vi "Sequence.vi"() -> ()   [LabVIEW 2016]
uses:
  PID2ChanGlobals.vi
  Globals/LJ_Handles_Global.vi
  <vilib>/Utility/file.llb/Write Delimited Spreadsheet (DBL).vi
panel:
  out "path":path=path "_run0.txt"
  in  "Run":dbl=102.0
  out "Recording Time":dbl=30.0
  out "Measured Ratio":dbl[](graph)
  in  "file path (dialog if empty)":path=path "E:/maggot images/Jacob/20170911/Fluorescein_Test_Step2a_run"
  in  "Add Ctrl?":bool
  in  "Setpoint":dbl[](array[numeric])=[0.9, 0.8, 0.7, 0.6, 0.5, 0.4, 0.3, 0.2, 0.1]
  in  "Time":dbl[](array[numeric])=[30.0, 30.0, 30.0, 30.0, 30.0, 30.0, 30.0, 30.0, 30.0]
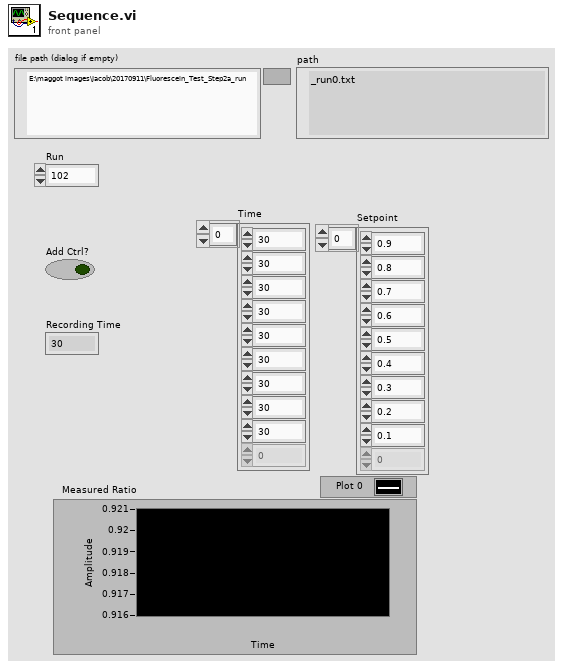
[diagram p1: front panel]
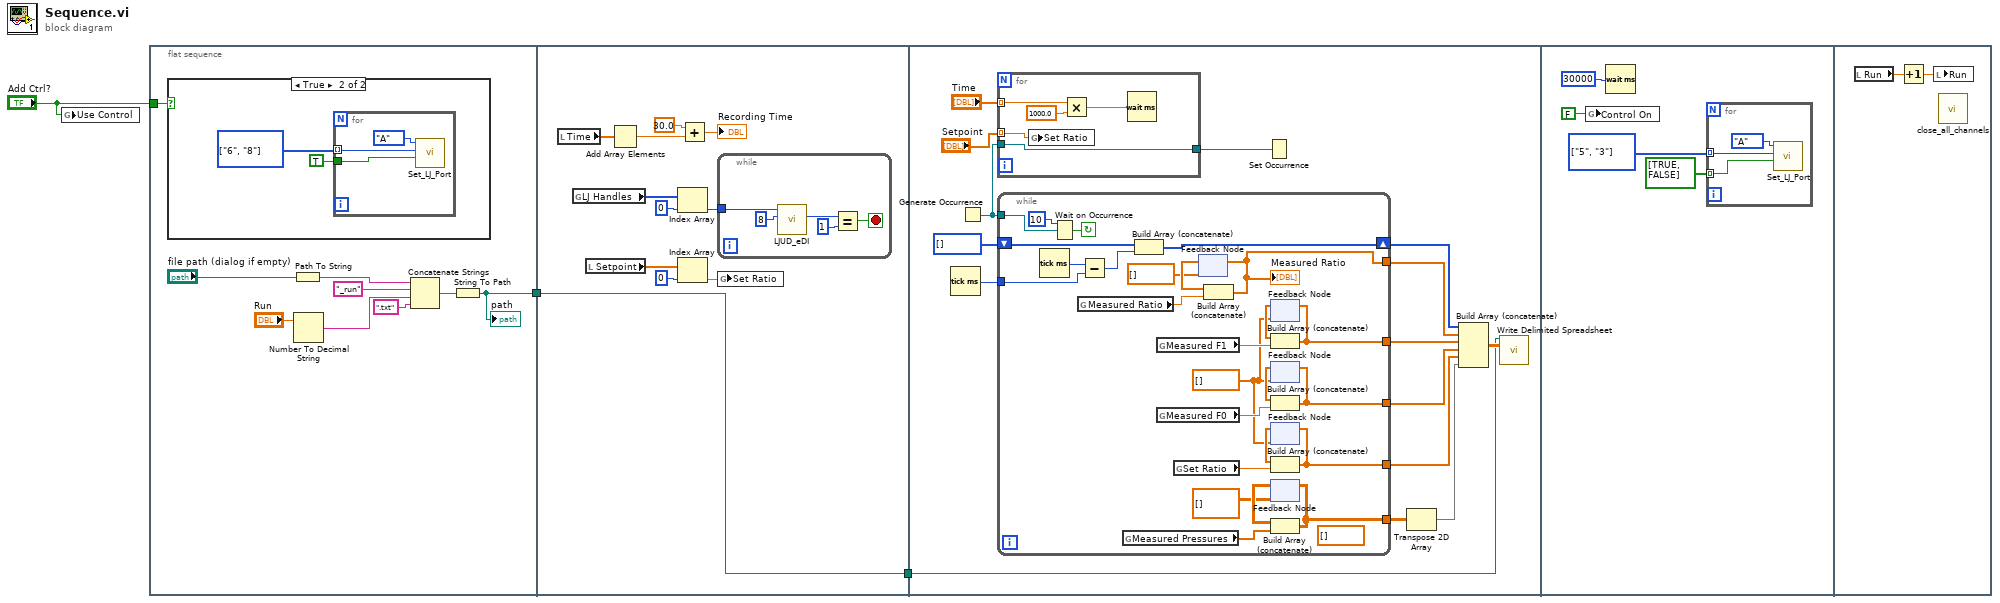
[diagram p0: block diagram]
diagram:
  n1 = global write "PID2ChanGlobals.vi" "Use Control"("Add Ctrl?") -> ()
  n2 = flat-sequence {
    tunnel: "Add Ctrl?" -> [w12]
    tunnel: [w4] -> w1
    tunnel: [w18] -> w2
    tunnel: w1 -> [w18]
    tunnel: w2 -> [w36]
    frame #0 {
      n3 = case shown="True" w12 {
        frame False {
        }
        frame True {
          w13 = enum16{"1", "2", "3", "4", "5", "6", "7", "8"}[] [enum."6", enum."8"] items=["1", "2", "3", "4", "5", "6", "7", "8"]
          n4 = for {
            tunnel: TRUE ("State") -> [w17]
            tunnel: w13 -> [w16] mode=indexing
            n5 = call "Set_LJ_Port.vi"("State"=w17, "Channel"=w16, "Flowboard"=enum16{"A", "B", "C"}."A") -> ()  [unwired: 8 in, 1 out]
          }
        }
      }
      n6 = Path To String(path="file path (dialog if empty)") -> (string=w7:string)
      n7 = Number To Decimal String(number="Run") -> (decimal integer string=w8:string)  [unwired: 1 in]
      n8 = Concatenate Strings(w7, "_run" ("string"), w8, ".txt" ("string")) -> (w5:string)
      n9 = String To Path(string=w5) -> (path=w4:path)
      "path" <- w4
    }
    frame #1 {
      n10 = local read "Time"() -> (w22:dbl[])
      n11 = global read "LJ_Handles_Global.vi" "LJ Handles"() -> (w27:i32[])
      n12 = local read "Setpoint"() -> (w24:dbl[])
      n13 = Add Array Elements(numeric array=w22) -> (sum=w21:dbl)
      n14 = Index Array(array=w27, index=0) -> (element=w26:i32)
      n15 = Index Array(array=w24, index=0) -> (element=w23:dbl)
      n16 = Add(x=30.0, y=w21) -> (x+y=→"Recording Time":dbl)
      n17 = while {
        tunnel: w26 -> [w33]
        stop <- w29 stop-if-true
        n18 = call "LJUD_eDI.vi"("Channel"=8, "Handle In"=w33) -> ("State"=w31:i32)  [unwired: 7 in, 2 out]
        n19 = Equal?(x=w31, y=1) -> (x = y?=w29:bool)
      }
      n20 = global write "PID2ChanGlobals.vi" "Set Ratio"(w23) -> ()
    }
    frame #2 {
      n21 = Tick Count (ms)() -> (millisecond timer value=w43:u32)
      n22 = Generate Occurrence() -> (w45:refnum<k4>)
      n23 = for {
        tunnel: "Time" -> [w76] mode=indexing
        tunnel: "Setpoint" -> [w78] mode=indexing
        tunnel: w45 -> [w79]
        tunnel: [w79] -> w46
        n24 = global write "PID2ChanGlobals.vi" "Set Ratio"(w78) -> ()
        n25 = Multiply(x=w76, y=1000.0) -> (x*y=w75:dbl)
        n26 = Wait (ms)(milliseconds to wait=w75) -> ()  [unwired: 1 out]
      }
      n27 = while {
        tunnel: w45 -> [w73]
        tunnel: [w70] -> w42
        tunnel: w43 -> [w68]
        tunnel: [w62] -> w40
        tunnel: [w59] -> w39
        tunnel: [w56] -> w38
        tunnel: [w53] -> w37
        shift-right: [w69] -> w41
        shift-left: u32[] [] -> [w50]
        stop <- w74 continue-if-true
        (unwired) dbl[] []
        w52 = dbl[] []
        n28 = Tick Count (ms)() -> (millisecond timer value=w67:u32)
        n29 = Wait on Occurrence(2:w73, 3:10 ("ms timeout (-1)")) -> (0:w74:bool)  [unwired: 1 in]
        n30 = global read "PID2ChanGlobals.vi" "Measured Ratio"() -> (w71:dbl)
        n31 = Subtract(x=w67, y=w68) -> (x-y=w66:u32)
        n32 = global read "PID2ChanGlobals.vi" "Measured Pressures"() -> (w55:dbl[])
        n33 = Build Array (concatenate)(w50, w66) -> (w69:u32[])
        n34 = global read "PID2ChanGlobals.vi" "Measured F1"() -> (w64:dbl)
        n35 = global read "PID2ChanGlobals.vi" "Measured F0"() -> (w61:dbl)
        n36 = global read "PID2ChanGlobals.vi" "Set Ratio"() -> (w58:dbl)
        n37 = feedback #1(dbl[] []) -> (w72:dbl[])
        n38 = Build Array (concatenate)(w72, w71) -> (w70:dbl[])
        "Measured Ratio" <- w70
        n39 = feedback-in #1(w70) -> ()
        n40 = feedback #2(w52) -> (w63:dbl[])
        n41 = Build Array (concatenate)(w63, w64) -> (w62:dbl[])
        n42 = feedback-in #2(w62) -> ()
        n43 = feedback #3(w52) -> (w60:dbl[])
        n44 = Build Array (concatenate)(w60, w61) -> (w59:dbl[])
        n45 = feedback-in #3(w59) -> ()
        n46 = feedback #4(w52) -> (w57:dbl[])
        n47 = Build Array (concatenate)(w57, w58) -> (w56:dbl[])
        n48 = feedback-in #4(w56) -> ()
        n49 = feedback #5(dbl[][] []) -> (w54:dbl[][])
        n50 = Build Array (concatenate)(w54, w55) -> (w53:dbl[][])
        n51 = feedback-in #5(w53) -> ()
      }
      n52 = Set Occurrence(w46) -> ()
      n53 = Transpose 2D Array(2D array=w37) -> (transposed array=w35:dbl[][])
      n54 = Build Array (concatenate)(w41, w42, w40, w39, w38, w35) -> (w44:dbl[][])
      n55 = call-poly <vilib>:"Write Delimited Spreadsheet.vi"("file path (dialog if empty)"=w36, "2D data"=w44) -> ()  [unwired: 12 in, 2 out]
    }
    frame #3 {
      w83 = enum16{"1", "2", "3", "4", "5", "6", "7", "8"}[] [enum."5", enum."3"] items=["1", "2", "3", "4", "5", "6", "7", "8"]
      n56 = global write "PID2ChanGlobals.vi" "Control On"(FALSE ("Control On")) -> ()
      n57 = Wait (ms)(milliseconds to wait=u32 30000) -> ()  [unwired: 1 out]
      n58 = for {
        tunnel: bool[] [TRUE, FALSE] -> [w86] mode=indexing
        tunnel: w83 -> [w85] mode=indexing
        n59 = call "Set_LJ_Port.vi"("State"=w86, "Channel"=w85, "Flowboard"=enum16{"A", "B", "C"}."A") -> ()  [unwired: 8 in, 1 out]
      }
    }
    frame #4 {
      n60 = local read "Run"() -> (w88:dbl)
      n61 = Increment(x=w88) -> (x+1=w87:dbl)
      n62 = local write "Run"(w87) -> ()
      n63 = call "close_all_channels.vi"() -> ()  [unwired: 12 in]
    }
  }
